vi "Select values for chosen axes.vi"(2 "Queried axes":string[](array[string]), 3 "Values":dbl[](array[numeric]) format="%.6f", 4 "Axes subset":string[](array[string]), 6 "Bool. Values":bool[](array[boolean]), 7 "String values":string[](array[string])) -> (14 "Values subset":dbl[](array[numeric]) format="%.6f", 15 "Bool. Values subset":bool[](array[boolean]), 16 "String values subset":string[](array[string]), 17 "Axes subset out":string[](array[string]))   [LabVIEW 2020]
doc: "This VI returns only values for the given axes subset."
panel:
  # "This vi returns only values for the given axes subset."
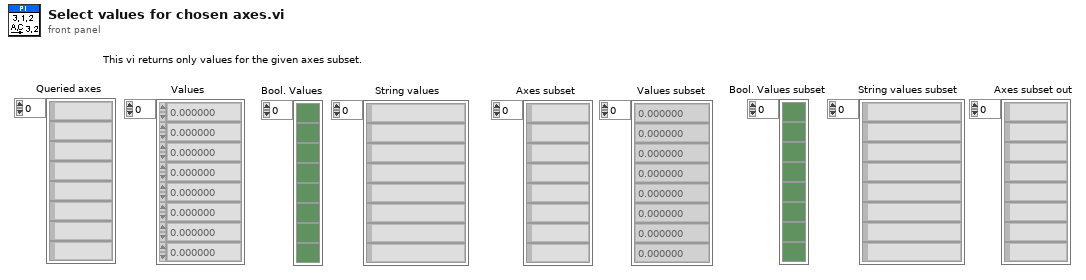
[diagram p1: front panel]
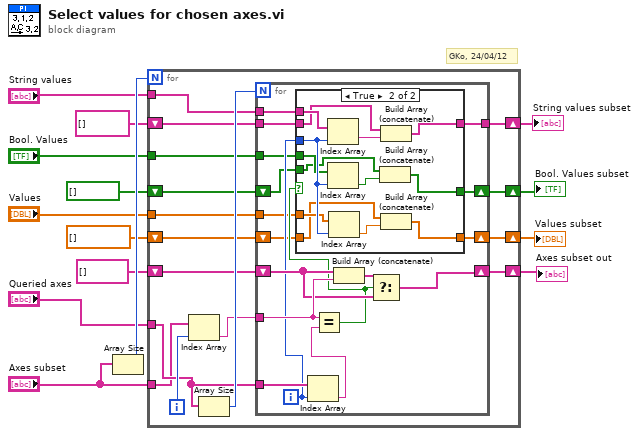
[diagram p0: block diagram]
diagram:
  # "GKo, 24/04/12"
  n1 = Array Size(array="Axes subset") -> (size(s)=w14:i32)
  n2 = for {
    N: w14 -> [_]
    shift-right: [w17] -> w13
    shift-left: dbl[] [] -> [w18]
    tunnel: "Queried axes" -> [w16]
    tunnel: "Axes subset" -> [w15]
    tunnel: "Values" -> [w23]
    tunnel: "String values" -> [w25]
    tunnel: "Bool. Values" -> [w24]
    shift-right: [w21] -> w5
    shift-left: string[] [] -> [w22]
    shift-right: [w19] -> w4
    shift-left: bool[] [] -> [w20]
    shift-right: [w27] -> w2
    shift-left: string[] [] -> [w26]
    i -> [w28]
    n3 = Index Array(array=w15, index=w28) -> (element=w29:string)
    n4 = Array Size(array=w16) -> (size(s)=w30:i32)
    n5 = for {
      N: w30 -> [_]
      tunnel: w29 -> [w44]
      tunnel: w16 -> [w47]
      shift-right: [w45] -> w27
      shift-left: w26 -> [w43]
      tunnel: w25 -> [w40]
      tunnel: w24 -> [w38]
      tunnel: w23 -> [w37]
      tunnel: w22 -> [w36]
      tunnel: [w35] -> w21
      shift-right: [w31] -> w17
      shift-left: w18 -> [w32]
      shift-right: [w33] -> w19
      shift-left: w20 -> [w34]
      i -> [w39]
      n6 = Index Array(array=w47, index=w39) -> (element=w46:string)
      n7 = Equal?(x=w44, y=w46) -> (x = y?=w41:bool)
      n8 = case shown="True" w41 {
        tunnel: w40 -> [_ w63]
        tunnel: w39 -> [_ w62]
        tunnel: w38 -> [_ w61]
        tunnel: w37 -> [_ w60]
        tunnel: w36 -> [w50 w58]
        tunnel: [w50 w57] -> w35
        tunnel: w34 -> [w49 w56]
        tunnel: [w49 w54] -> w33
        tunnel: w32 -> [w48 w53]
        tunnel: [w48 w51] -> w31
        frame False {
        }
        frame True {
          n9 = Index Array(array=w63, index=w62) -> (element=w59:string)
          n10 = Index Array(array=w61, index=w62) -> (element=w55:bool)
          n11 = Index Array(array=w60, index=w62) -> (element=w52:dbl)
          n12 = Build Array (concatenate)(w56, w55) -> (w54:bool[])
          n13 = Build Array (concatenate)(w58, w59) -> (w57:string[])
          n14 = Build Array (concatenate)(w53, w52) -> (w51:dbl[])
        }
      }
      n15 = Build Array (concatenate)(w43, w44) -> (w42:string[])
      n16 = Select(t=w42, s=w41, f=w43) -> (s? t:f=w45:string[])
    }
  }
  "Values subset" <- w13
  "Bool. Values subset" <- w4
  "String values subset" <- w5
  "Axes subset out" <- w2
